vi "系统变量.vi"() -> ()   [LabVIEW 2016]
panel:
  in  "运行模式":enum16{"维护模式", "常规模式", "应急模式", "质控模式"}(ring)
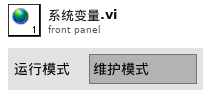
[diagram p1: front panel]
diagram:
